vi "JKISM++ Synchronized Call.vi"   [LabVIEW 2014, in "JKI State Machine++.lvlib"]
doc: "VI snippet for dropping sync call template code from LabVIEW Quick Drop.\n\n<b>Inputs:</b>\n - N/A\n -\n<b>Outputs:</b>\n - N/A"
uses:
  JKI State Machine++.lvlib
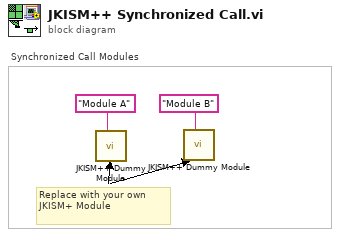
[diagram p0: block diagram]
diagram:
  # "Synchronized Call Modules"
  # "Replace with your own JKISM+ Module"
  n1 = call "JKISM++ Dummy Module.vi"("Name(\"\" to use uuid)"="Module A" ("Name(\"\" to use uuid)")) -> ()  [unwired: 11 in]
  n2 = call "JKISM++ Dummy Module.vi"("Name(\"\" to use uuid)"="Module B" ("Name(\"\" to use uuid)")) -> ()  [unwired: 11 in]
